vi "List Linked List Roots.vi"(8 "error in (no error)":errorcluster, 11 "Linked List in":refnum<class "Linked List.lvclass">) -> (0 "error out":errorcluster, 1 "Root Names":string[](array[string]), 2 "Root IDs":string[](array[string]), 3 "Linked List out":refnum<class "Linked List.lvclass">)   [LabVIEW 2020, in "Linked Lists.lvlib" / "Linked List.lvclass"]
uses:
  <vilib>/gpm_packages/@cs/linked-list/Source/Linked List/Linked List/Linked List.lvclass
  <vilib>/gpm_packages/@cs/linked-list/Source/Linked List/Linked List/Linked List.lvclass/Linked List.ctl
  <vilib>/gpm_packages/@cs/lookup-table/Source/LookupTable/LookupTable.lvclass/LookupTable.ctl
  <vilib>/gpm_packages/@cs/lookup-table/Source/LookupTable/Read Table Reference.vi
  <vilib>/gpm_packages/@cs/lookup-table/Source/LookupTable/LookupTable.lvclass
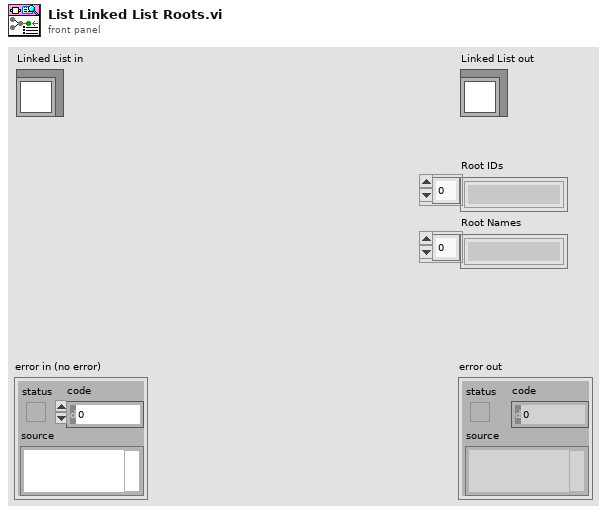
[diagram p1: front panel]
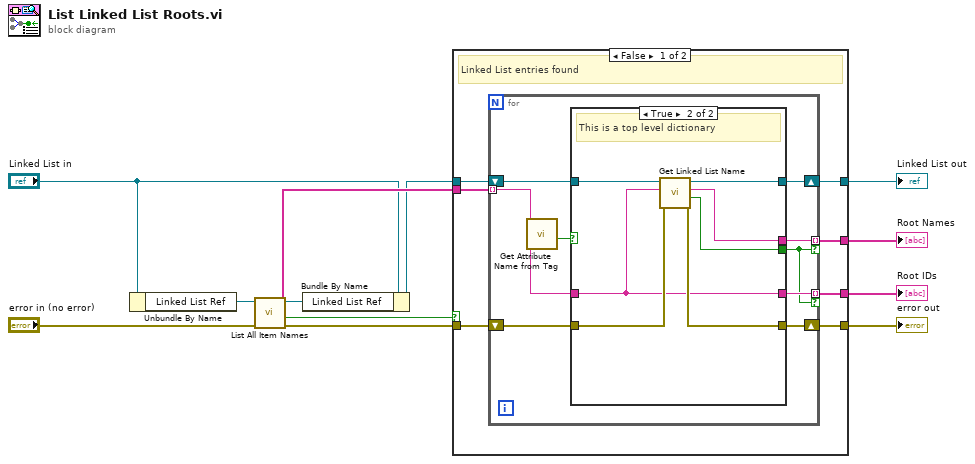
[diagram p0: block diagram]
diagram:
  n1 = Unbundle By Name("Linked List in") -> ("Linked List Ref"=w12:refnum<data-value>)
  n2 = call <vilib>:"List All Item Names.vi"("error in (no error)"="error in (no error)", "LookupTable Reference"=w12) -> ("error out"=w8:errorcluster, "None Found?"=w9:bool, "All Items"=w7:string[], "LookupTable Reference Out"=w10:refnum<data-value>)  [unwired: 6 in]
  n3 = Bundle By Name(cluster="Linked List in", "Linked List Ref"=w10) -> (w5:refnum<class "Linked List.lvclass">)
  n4 = case shown="False" w9 {
    tunnel: w8 -> [w16 w38]
    tunnel: w7 -> [w17 _]
    tunnel: w5 -> [w19 w39]
    tunnel: [w18 w39] -> w4
    tunnel: [w15 w38] -> w3
    tunnel: [w14 _] -> w2
    tunnel: [w13 _] -> w1
    frame False {
      # "Linked List entries found"
      n5 = for {
        shift-right: [w28] -> w18
        shift-left: w19 -> [w27]
        tunnel: w17 -> [w25] mode=indexing
        shift-right: [w23] -> w15
        shift-left: w16 -> [w24]
        tunnel: [w22] -> w14 mode=indexing if=w20
        tunnel: [w21] -> w13 mode=indexing if=w20
        n6 = call <vilib>:"Get Attribute Name from Tag.vi"("Tag"=w25) -> ("Linked List"=w26:bool)  [unwired: 8 in, 2 out]
        n7 = case shown="True" w26 {
          tunnel: [w30 w36] -> w28
          tunnel: w27 -> [w30 w37]
          tunnel: w25 -> [_ w33]
          tunnel: w24 -> [w29 w35]
          tunnel: [w29 w34] -> w23
          tunnel: [_ w33] -> w22
          tunnel: [_ w32] -> w21
          tunnel: [_ w31] -> w20
          frame False {
            # "This is not a top level dictioary"
          }
          frame True {
            # "This is a top level dictionary"
            n8 = call-dynamic "Get Linked List Name.vi"("error in (no error)"=w35, "Unique ID"=w33, "Linked List in"=w37) -> ("error out"=w34:errorcluster, "I am Root?"=w31:bool, "Linked List Name"=w32:string, "Linked List out"=w36:refnum<class "Linked List.lvclass">)  [unwired: 5 in]
          }
        }
      }
    }
    frame True {
      # "No dictionary entries found"
    }
  }
  "error out" <- w3
  "Linked List out" <- w4
  "Root Names" <- w1
  "Root IDs" <- w2
